vi "GE 5565PIORC.DMA.Create Transfer (Scatter-Gather).vi"(8 "error in (no error)":errorcluster, 9 "RFM offset":u32, 10 "Block Descriptors":T2[](array[typedef]) {"descriptor params"."data ptr (lower)" format="%.0x"; "descriptor params"."data ptr (upper)" format="%.0x"; "descriptor params"."data size" format="%.0x"; "descriptor params"."next descriptor ptr" format="%.0x"; "descriptor size" format="%08x"; "descriptor ptr (RFM)" format="%08x"; "descriptor ptr (VISA)" format="%08x"}, 11 "GE 5565PIORC in":refnum<class "GE 5565PIORC.lvclass">) -> (0 "error out":errorcluster, 1 "transfer size (bytes)":u32, 2 "DMA Transfer Spec":T1 {"Block Descriptors"."descriptor params"."data ptr (lower)" format="%.0x"; "Block Descriptors"."descriptor params"."data ptr (upper)" format="%.0x"; "Block Descriptors"."descriptor params"."data size" format="%.0x"; "Block Descriptors"."descriptor params"."next descriptor ptr" format="%.0x"; "Block Descriptors"."descriptor size" format="%08x"; "Block Descriptors"."descriptor ptr (RFM)" format="%08x"; "Block Descriptors"."descriptor ptr (VISA)" format="%08x"; "RFM offset" format="%08x"}, 3 "GE 5565PIORC out":refnum<class "GE 5565PIORC.lvclass">)   [LabVIEW 2016, in "GE 5565PIORC.lvclass"]
doc: "Creates a <B>DMA Transfer Spec</B> which associates a series of <B>Block Descriptors</B> to an offset in Reflective Memory."
uses:
  GE 5565PIORC.lvclass
  Typedefs/GE 5565PIORC.Typedef.DMA Block Descriptor.ctl
  Typedefs/GE 5565PIORC.Typedef.DMA Block Descriptor Params.ctl
  Typedefs/GE 5565PIORC.Typedef.DMA Transfer Spec.ctl
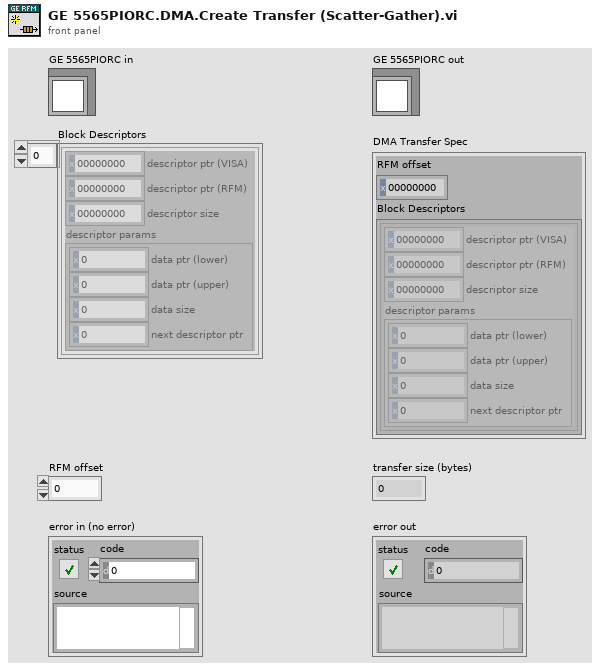
[diagram p1: front panel]
types:
  T1 = typedef "GE 5565PIORC.lvclass/GE 5565PIORC.Typedef.DMA Transfer Spec.ctl" = cluster{"RFM offset":u32, "Block Descriptors":T2[]}
  T2 = typedef "GE 5565PIORC.lvclass/GE 5565PIORC.Typedef.DMA Block Descriptor.ctl" = cluster{"descriptor ptr (VISA)":u32, "descriptor ptr (RFM)":u32, "descriptor size":u32, "descriptor params":T3}
  T3 = typedef "GE 5565PIORC.lvclass/GE 5565PIORC.Typedef.DMA Block Descriptor Params.ctl" = cluster{"data ptr (lower)":u32, "data ptr (upper)":u32, "data size":u32, "next descriptor ptr":u32}
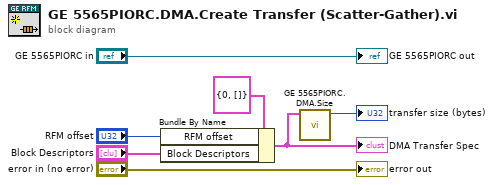
[diagram p0: block diagram]
diagram:
  n1 = Bundle By Name(cluster=T1 {"RFM offset"=0, "Block Descriptors"=[]} ("DMA Transfer Spec"), "RFM offset"="RFM offset", "Block Descriptors"="Block Descriptors") -> (w2:T1)
  "DMA Transfer Spec" <- w2
  n2 = call "GE 5565PIORC.DMA.Size.vi"("DMA Transfer Spec in"=w2) -> ("transfer size (bytes)"=→"transfer size (bytes)":u32)  [unwired: 10 in]
  "GE 5565PIORC out" <- "GE 5565PIORC in"
  "error out" <- "error in (no error)"
